vi "Read Waveforms (Single).vi"(7 "Bind Source Channel (2: None)":i32(ring)=2 items=["Sub Source 0", "Sub Source 1", "None"], 8 "error in (no error)":errorcluster, 9 "Timeout (10000 ms)":u32=10000, 10 "Source Channel (0: Channel 1)":i32(ring) items=["Channel 1"=0, "Channel 2"=1, "Channel 3"=2, "Channel 4"=3, "Waveform Memory 1"=5, "Waveform Memory 2"=6, "Serial Bus 1"=7, "Serial Bus 2"=8, "Digital Bus Low"=9, "Digital Bus High "=10, "Digital Bus 1"=11, "Digital Bus 2"=12, "External"=29, "Function 1"=32, "Function 2"=33, "Function 3"=34, "Function 4"=35, "Math 1"=36, "Math 2"=37, "Math 3"=38, "Math 4"=39, "FFT"=40, "Analog Bus"=41], 11 "VISA resource name":refnum<visa-resource-name>) -> (0 "error out":errorcluster, 2 "Waveform Data":waveform(dbl)(graph), 3 "VISA resource name out":refnum<visa-resource-name>)   [LabVIEW 2016, in "Agilent 2000 3000 X-Series.lvlib"]
doc: "Initiates an acquisition on all channels that you enabled with the Configure Channel VI. The VI waits for the acquisition to complete and returns the waveform for the <B>Source Channel</B> you specified. If the oscilloscope did not complete the acquisition within the time period you specify with the <B>Timeout</B> control, the VI returns a timeout error. A common cause for a timeout error is the acquisition was not triggered. For example, the trigger level is out of range of the waveform.\n\nCall the Fetch Waveform VI to obtain the waveforms for each of the remaining enabled <B>Source Channels</B> without initiating another acquisition.\n\n<B>Note(s):</B> \nIf your instrument does not support auto compensation for probe attenuation, you may need to adjust the scaling of the Waveform Data accordingly. This is handled automatically in the <B>Configure Channel</B> VI or can be done manually by multiplying the <B>Waveform Data</B> by the probe attenuation."
uses:
  Agilent 2000 3000 X-Series.lvlib
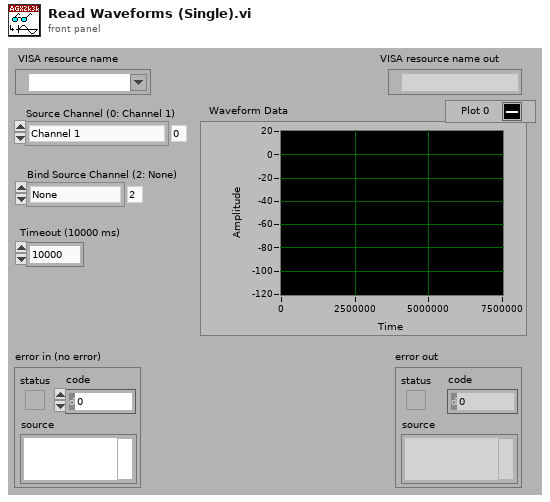
[diagram p1: front panel]
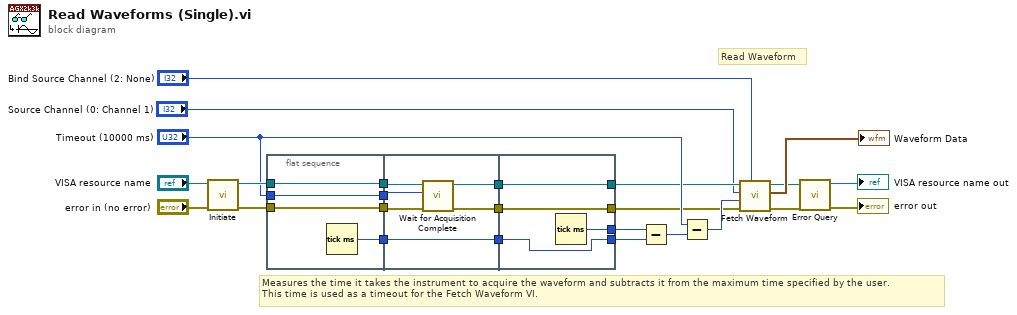
[diagram p0: block diagram]
diagram:
  # "Measures the time it takes the instrument to acquire the waveform and subtracts it from the maximum time specified by the user.\nThis time is used as a timeout for the Fetch Waveform VI."
  # "Read Waveform"
  n1 = call "Initiate.vi"("error in (no error)"="error in (no error)", "VISA resource name"="VISA resource name") -> ("error out"=w20:errorcluster, "VISA resource name out"=w21:refnum<visa-resource-name>)  [unwired: 8 out]
  n2 = flat-sequence {
    tunnel: w21 -> [w28]
    tunnel: [w28] -> w8
    tunnel: w20 -> [w27]
    tunnel: [w27] -> w7
    tunnel: "Timeout (10000 ms)" -> [w26]
    tunnel: [w26] -> w6
    tunnel: [w29] -> w5
    tunnel: w8 -> [w35]
    tunnel: [w33] -> w4
    tunnel: w7 -> [w34]
    tunnel: [w32] -> w3
    tunnel: w6 -> [w31]
    tunnel: w5 -> [w30]
    tunnel: [w30] -> w2
    tunnel: [w38] -> w16
    tunnel: w4 -> [w38]
    tunnel: [w37] -> w17
    tunnel: w3 -> [w37]
    tunnel: [w36] -> w25
    tunnel: w2 -> [w36]
    tunnel: [w39] -> w24
    frame #0 {
      n3 = Tick Count (ms)() -> (millisecond timer value=w29:u32)
    }
    frame #1 {
      n4 = call "Wait for Acquisition Complete.vi"("error in (no error)"=w34, "Maximum Time (10000)"=w31, "VISA resource name"=w35) -> ("error out"=w32:errorcluster, "VISA resource name out"=w33:refnum<visa-resource-name>)  [unwired: 7 out]
    }
    frame #2 {
      n5 = Tick Count (ms)() -> (millisecond timer value=w39:u32)
    }
  }
  n6 = Subtract(x=w24, y=w25) -> (x-y=w9:u32)
  n7 = Subtract(x="Timeout (10000 ms)", y=w9) -> (x-y=w18:u32)
  n8 = call "Fetch Waveform.vi"("Bind Source Channel (2: None)"="Bind Source Channel (2: None)", "error in (no error)"=w17, "Timeout (10000)"=w18, "Source Channel (0: Channel 1)"="Source Channel (0: Channel 1)", "VISA resource name"=w16) -> ("error out"=w11:errorcluster, "Waveform Data"=→"Waveform Data":waveform(dbl), "VISA resource name out"=w13:refnum<visa-resource-name>)  [unwired: 4 out]
  n9 = call "Error Query.vi"("error in (no error)"=w11, "VISA resource name"=w13) -> ("error out"=→"error out":errorcluster, "VISA resource name out"=→"VISA resource name out":refnum<visa-resource-name>)  [unwired: 8 out]
